vi "solar Setup.vi"(8 "error in (no error)":errorcluster, 11 "solar in":refnum<class "solar.lvclass">) -> (0 "error out":errorcluster, 3 "solar out":refnum<class "solar.lvclass">)   [LabVIEW 2018, in "solar.lvclass"]
doc: "Setup target references"
uses:
  solar.lvclass
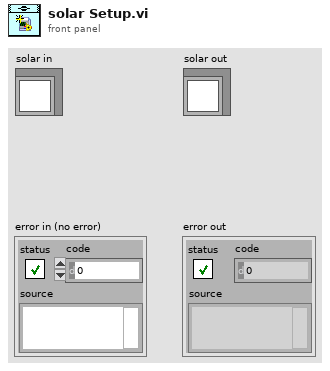
[diagram p1: front panel]
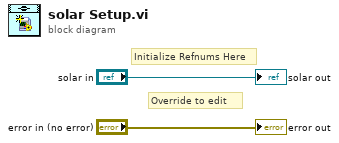
[diagram p0: block diagram]
diagram:
  # "Initialize Refnums Here"
  # "Override to edit"
  "error out" <- "error in (no error)"
  "solar out" <- "solar in"
